vi "torres hanoi.vi"() -> ()   [LabVIEW 2020]
uses:
  <vilib>/Utility/miscctls.llb/LVPoint32TypeDef.ctl
  <vilib>/Utility/miscctls.llb/LVPositionTypeDef.ctl
  <vilib>/Utility/miscctls.llb/LVBoundsTypeDef.ctl
panel:
  out "Position 1":T1
  out "Position 2":T1
  out "Position 3":T1
  out "Position 4":T1
  out "Position 5":T1
  out "Position":T1
  in  "seleccione  numero de discos":u16(ring) items=["3"=3, "4"=4, "5"=5]
  out "Coords":T2
  in  "?":bool
  out "disco5":bool
  out "disco4":bool
  out "disco3":bool
  out "disco2":bool
  out "disco1":bool
  out "final":bool
  out "medio":bool
  out "inicio":bool
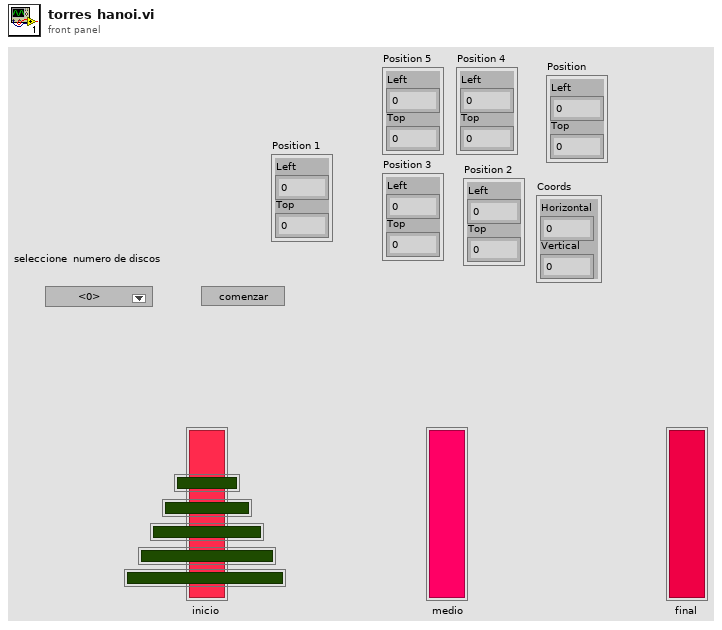
[diagram p1: front panel]
types:
  T1 = typedef "LVPositionTypeDef.ctl" = cluster{"Left":i32, "Top":i32}
  T2 = typedef "LVPoint32TypeDef.ctl" = cluster{"Horizontal":i32, "Vertical":i32}
  T3 = typedef "LVBoundsTypeDef.ctl" = cluster{"Width":u32, "Height":u32}
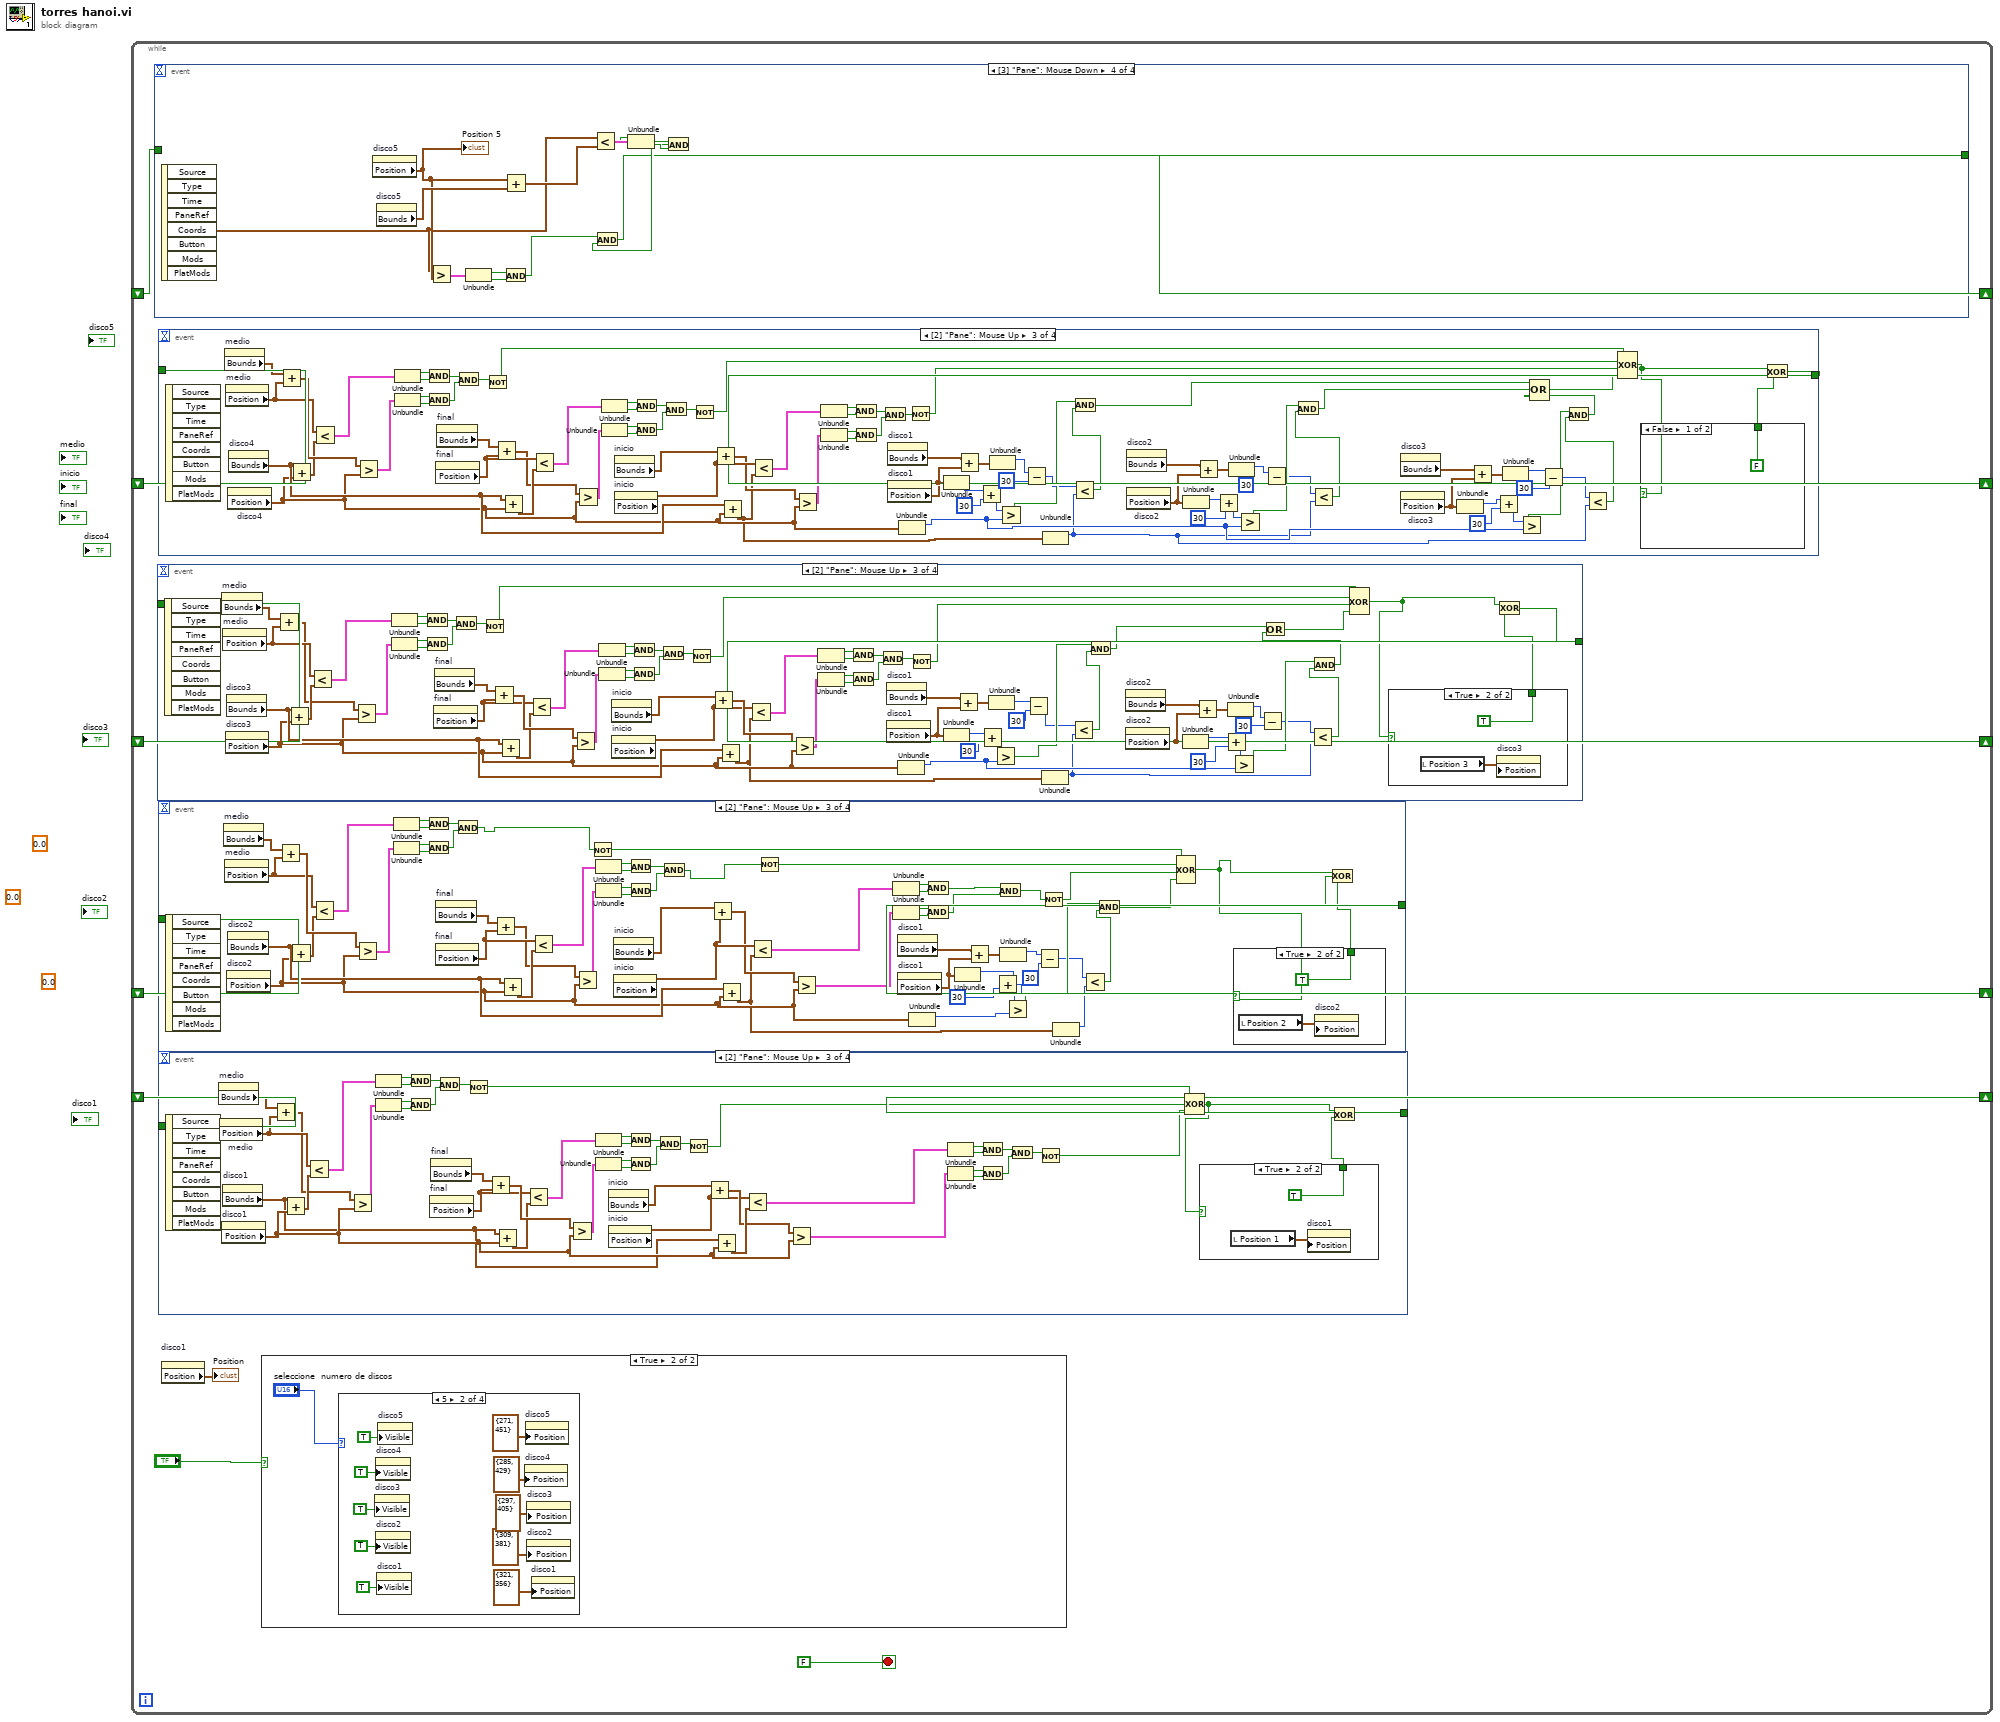
[diagram p0: block diagram]
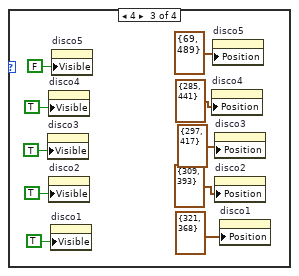
[diagram p4: hidden frame]
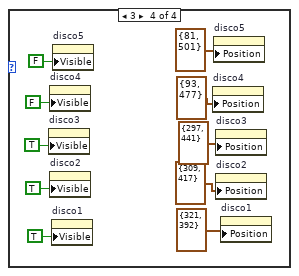
[diagram p5: hidden frame]
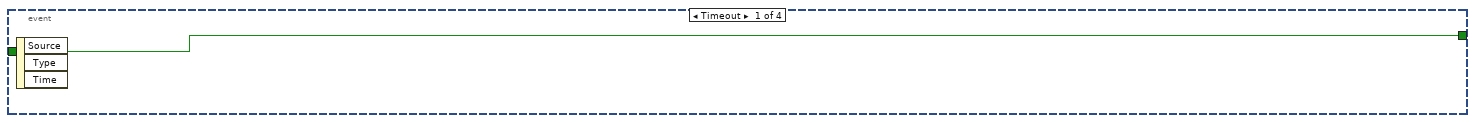
[diagram p6: hidden frame]
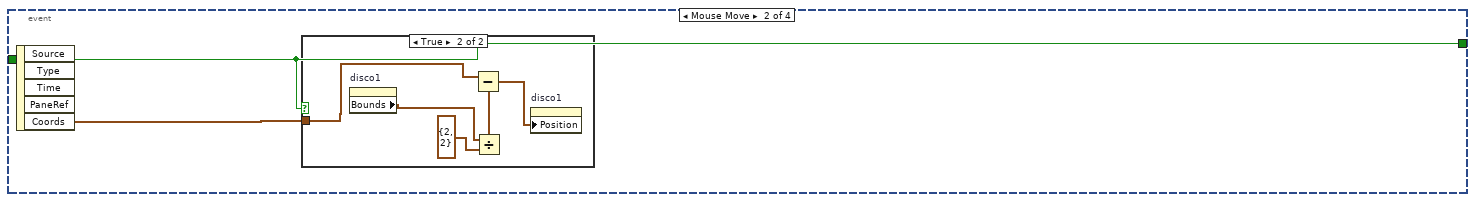
[diagram p7: hidden frame]
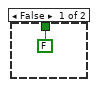
[diagram p9: hidden frame]
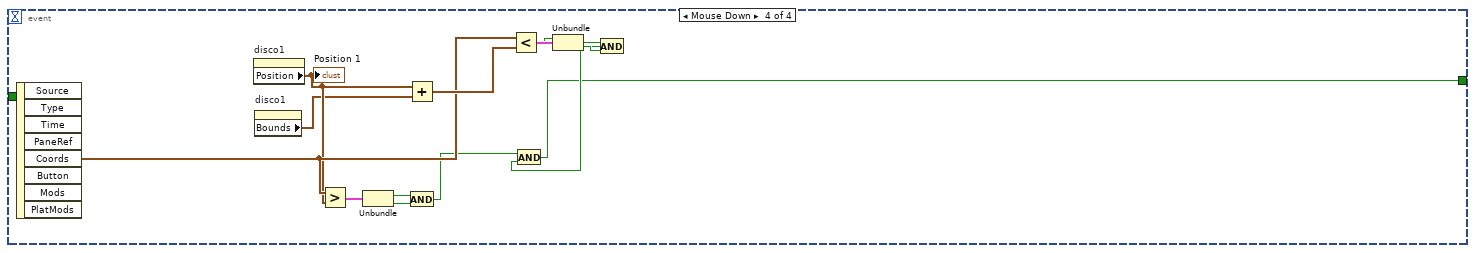
[diagram p10: hidden frame]
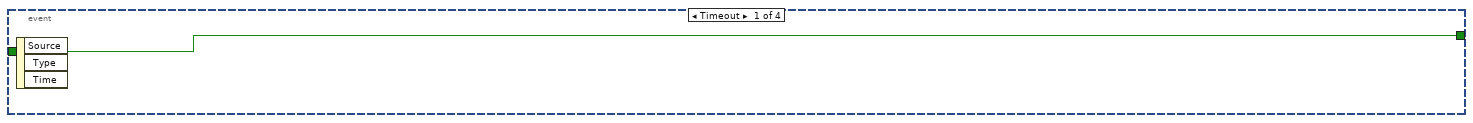
[diagram p11: hidden frame]
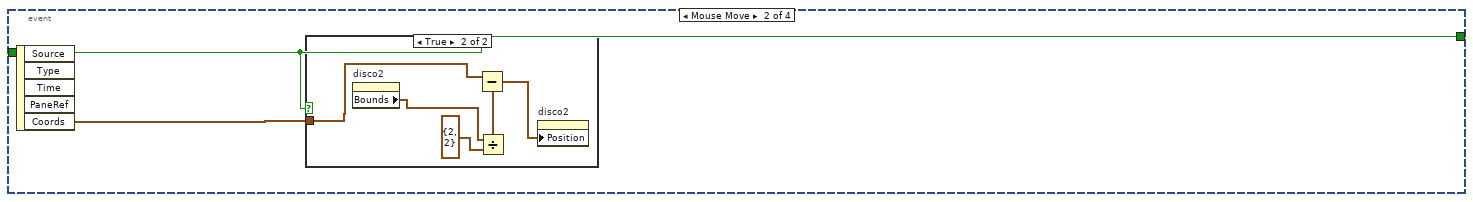
[diagram p12: hidden frame]
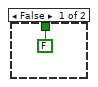
[diagram p14: hidden frame]
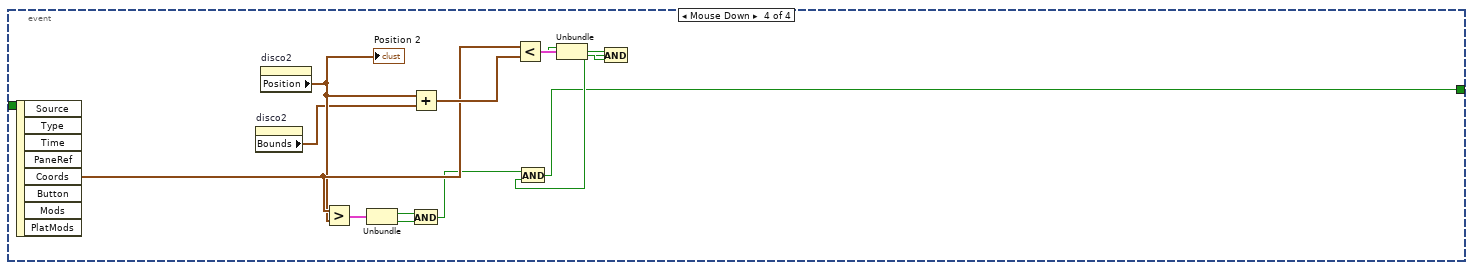
[diagram p15: hidden frame]
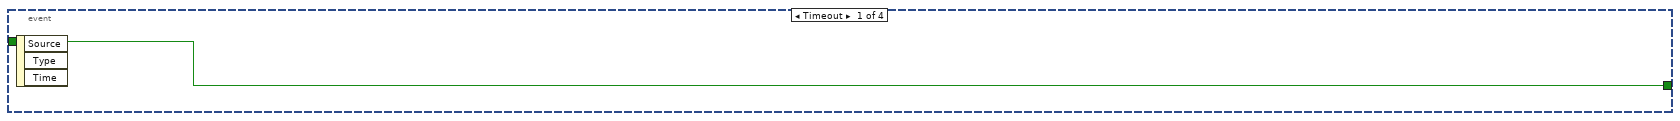
[diagram p16: hidden frame]
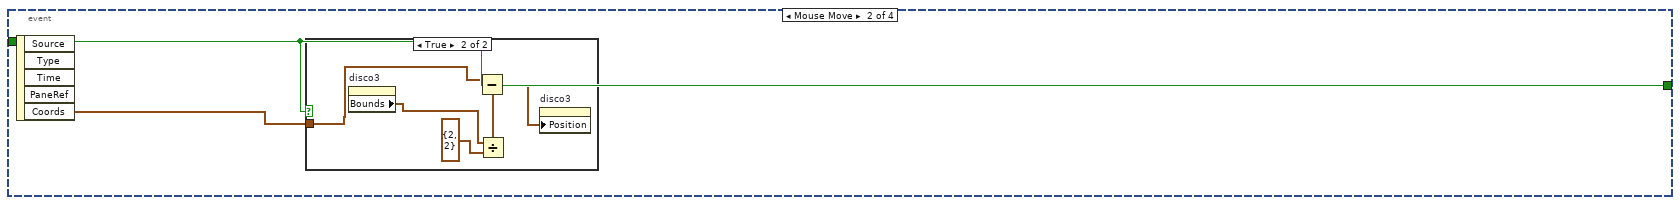
[diagram p17: hidden frame]
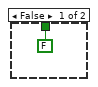
[diagram p19: hidden frame]
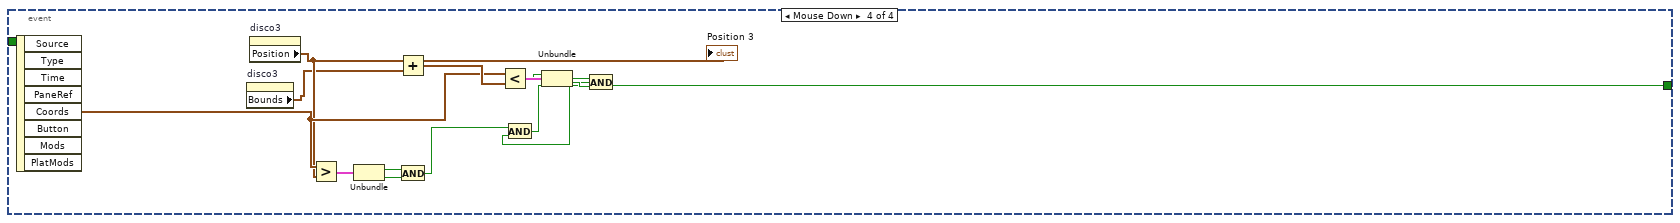
[diagram p20: hidden frame]
diagram:
  (unwired) 0.0 ("final b")
  (unwired) 0.0 ("inicio b")
  (unwired) 0.0 ("medio b")
  n1 = while {
    shift-right: [w11] -> _
    shift-left: _ -> [w12]
    shift-right: [w9] -> _
    shift-left: _ -> [w10]
    shift-right: [w7] -> _
    shift-left: _ -> [w8]
    shift-right: [w5] -> _
    shift-left: _ -> [w6]
    shift-right: [w3] -> _
    shift-left: _ -> [w4]
    stop <- FALSE stop-if-true
    n2 = event shown="[3] \"Pane\": Mouse Down" {
      selector: _ -> [_ _ _ _]
      dyn-events: _ -> [_ _ _ _]
      timeout: _ -> [_ _ _ _]
      tunnel: w12 -> [w409 w410 _ _]
      tunnel: [w409 w410 w470 w518] -> w11
      event Timeout {
        n3 = event-data() -> ()  [unwired: 1 in, 3 out]
      }
      event Mouse Move {
        n4 = event-data() -> ("Coords"=w411:T2)  [unwired: 1 in, 4 out]
        n5 = case shown="True" w410 {
          tunnel: w411 -> [_ w414]
          frame False {
          }
          frame True {
            n6 = property on="disco5" class="Bool (strict)"() -> ("Bounds"=w416:T3)  [unwired: 2 in, 2 out]
            n7 = Divide(x=w416, y=T3 {"Width"=2, "Height"=2}) -> (x/y=w413:cluster{"Width":dbl, "Height":dbl})
            n8 = Subtract(x=w414, y=w413) -> (x-y=w412:cluster{dbl, dbl})
            n9 = property on="disco5" class="Bool (strict)"("Position"=w412) -> ()  [unwired: 2 in, 2 out]
            "Coords" <- w414
          }
        }
      }
      event Mouse Up {
        n10 = event-data() -> ()  [unwired: 1 in, 8 out]
        n11 = property on="medio" class="Bool (strict)"() -> ("Bounds"=w505:T3)  [unwired: 2 in, 2 out]
        n12 = property on="medio" class="Bool (strict)"() -> ("Position"=w504:T1)  [unwired: 2 in, 2 out]
        n13 = property on="disco5" class="Bool (strict)"() -> ("Position"=w458:T1)  [unwired: 2 in, 2 out]
        n14 = property on="disco5" class="Bool (strict)"() -> ("Bounds"=w476:T3)  [unwired: 2 in, 2 out]
        n15 = Add(x=w505, y=w504) -> (x+y=w503:T3)
        n16 = Add(x=w476, y=w458) -> (x+y=w508:T3)
        n17 = Less?(x=w504, y=w508) -> (x < y?=w507:cluster{bool, bool})
        n18 = Greater?(x=w503, y=w458) -> (0:w506:cluster{bool, bool})
        n19 = Unbundle(w507) -> (w512:bool, w511:bool)
        n20 = Unbundle(w506) -> (w514:bool, w513:bool)
        n21 = And(x=w512, y=w511) -> (x .and. y?=w509:bool)
        n22 = And(x=w514, y=w513) -> (x .and. y?=w510:bool)
        n23 = property on="final" class="Bool (strict)"() -> ("Position"=w489:T1)  [unwired: 2 in, 2 out]
        n24 = property on="final" class="Bool (strict)"() -> ("Bounds"=w490:T3)  [unwired: 2 in, 2 out]
        n25 = And(x=w509, y=w510) -> (x .and. y?=w502:bool)
        n26 = Not(x=w502) -> (.not. x?=w473:bool)
        n27 = Add(x=w490, y=w489) -> (x+y=w500:T3)
        n28 = Add(x=w476, y=w458) -> (x+y=w497:T3)
        n29 = Less?(x=w489, y=w497) -> (x < y?=w498:cluster{bool, bool})
        n30 = Greater?(x=w500, y=w458) -> (0:w499:cluster{bool, bool})
        n31 = Unbundle(w498) -> (w493:bool, w494:bool)
        n32 = Unbundle(w499) -> (w491:bool, w492:bool)
        n33 = property on="inicio" class="Bool (strict)"() -> ("Bounds"=w478:T3)  [unwired: 2 in, 2 out]
        n34 = property on="inicio" class="Bool (strict)"() -> ("Position"=w477:T1)  [unwired: 2 in, 2 out]
        n35 = And(x=w493, y=w494) -> (x .and. y?=w496:bool)
        n36 = And(x=w491, y=w492) -> (x .and. y?=w495:bool)
        n37 = And(x=w496, y=w495) -> (x .and. y?=w501:bool)
        n38 = Not(x=w501) -> (.not. x?=w474:bool)
        n39 = Add(x=w478, y=w477) -> (x+y=w480:T3)
        n40 = Add(x=w476, y=w458) -> (x+y=w457:T3)
        n41 = Less?(x=w477, y=w457) -> (x < y?=w482:cluster{bool, bool})
        n42 = Greater?(x=w480, y=w458) -> (0:w481:cluster{bool, bool})
        n43 = Unbundle(w482) -> (w486:bool, w485:bool)
        n44 = Unbundle(w481) -> (w488:bool, w487:bool)
        n45 = property on="disco1" class="Bool (strict)"() -> ("Bounds"=w464:T3)  [unwired: 2 in, 2 out]
        n46 = property on="disco1" class="Bool (strict)"() -> ("Position"=w465:T1)  [unwired: 2 in, 2 out]
        n47 = Unbundle(w458) -> ("Left"=w447:i32)  [unwired: 1 out]
        n48 = And(x=w486, y=w485) -> (x .and. y?=w483:bool)
        n49 = And(x=w488, y=w487) -> (x .and. y?=w484:bool)
        n50 = And(x=w483, y=w484) -> (x .and. y?=w479:bool)
        n51 = Unbundle(w465) -> ("Left"=w445:i32)  [unwired: 1 out]
        n52 = Add(x=w464, y=w465) -> (x+y=w466:T3)
        n53 = Not(x=w479) -> (.not. x?=w475:bool)
        n54 = Add(x=w445, y=30) -> (x+y=w443:i32)
        n55 = Greater?(x=w443, y=w447) -> (0:w460:bool)
        n56 = Unbundle(w466) -> ("Width"=w442:u32)  [unwired: 1 out]
        n57 = Subtract(x=w442, y=u32 30) -> (x-y=w440:u32)
        n58 = Unbundle(w457) -> ("Width"=w446:u32)  [unwired: 1 out]
        n59 = Less?(x=w440, y=w446) -> (x < y?=w459:bool)
        n60 = And(x=w460, y=w459) -> (x .and. y?=w417:bool)
        n61 = property on="disco2" class="Bool (strict)"() -> ("Bounds"=w463:T3)  [unwired: 2 in, 2 out]
        n62 = property on="disco2" class="Bool (strict)"() -> ("Position"=w462:T1)  [unwired: 2 in, 2 out]
        n63 = Unbundle(w462) -> ("Left"=w438:i32)  [unwired: 1 out]
        n64 = Add(x=w463, y=w462) -> (x+y=w461:T3)
        n65 = Add(x=w438, y=30) -> (x+y=w439:i32)
        n66 = Unbundle(w461) -> ("Width"=w436:u32)  [unwired: 1 out]
        n67 = Greater?(x=w439, y=w447) -> (0:w456:bool)
        n68 = Subtract(x=w436, y=u32 30) -> (x-y=w435:u32)
        n69 = Less?(x=w435, y=w446) -> (x < y?=w455:bool)
        n70 = And(x=w456, y=w455) -> (x .and. y?=w418:bool)
        n71 = property on="disco3" class="Bool (strict)"() -> ("Bounds"=w467:T3)  [unwired: 2 in, 2 out]
        n72 = property on="disco3" class="Bool (strict)"() -> ("Position"=w468:T1)  [unwired: 2 in, 2 out]
        n73 = Unbundle(w468) -> ("Left"=w433:i32)  [unwired: 1 out]
        n74 = Add(x=w467, y=w468) -> (x+y=w469:T3)
        n75 = Add(x=w433, y=30) -> (x+y=w432:i32)
        n76 = Unbundle(w469) -> ("Width"=w430:u32)  [unwired: 1 out]
        n77 = Greater?(x=w432, y=w447) -> (0:w454:bool)
        n78 = Subtract(x=w430, y=u32 30) -> (x-y=w429:u32)
        n79 = Less?(x=w429, y=w446) -> (x < y?=w453:bool)
        n80 = And(x=w454, y=w453) -> (x .and. y?=w419:bool)
        n81 = property on="disco4" class="Bool (strict)"() -> ("Bounds"=w450:T3)  [unwired: 2 in, 2 out]
        n82 = property on="disco4" class="Bool (strict)"() -> ("Position"=w449:T1)  [unwired: 2 in, 2 out]
        n83 = Unbundle(w449) -> ("Left"=w427:i32)  [unwired: 1 out]
        n84 = Add(x=w450, y=w449) -> (x+y=w448:T3)
        n85 = Add(x=w427, y=30) -> (x+y=w426:i32)
        n86 = Greater?(x=w426, y=w447) -> (0:w451:bool)
        n87 = Unbundle(w448) -> ("Width"=w424:u32)  [unwired: 1 out]
        n88 = Subtract(x=w424, y=u32 30) -> (x-y=w422:u32)
        n89 = Less?(x=w422, y=w446) -> (x < y?=w452:bool)
        n90 = And(x=w451, y=w452) -> (x .and. y?=w420:bool)
        n91 = Compound Arithmetic op=OR(w417, w418, w419, w420) -> (w421:bool)
        n92 = Compound Arithmetic op=XOR(w473, w474, w475, w421) -> (w471:bool)
        n93 = case shown="True" w471 {
          tunnel: [FALSE ("Accepted?") TRUE ("Accepted?")] -> w472
          frame False {
          }
          frame True {
            n94 = local read "Position 5"() -> (w517:T1)
            n95 = property on="disco5" class="Bool (strict)"("Position"=w517) -> ()  [unwired: 2 in, 2 out]
          }
        }
        n96 = Exclusive Or(1:w472, 2:w471) -> (0:w470:bool)
      }
      event Mouse Down {
        n97 = event-data() -> ("Coords"=w527:T2)  [unwired: 1 in, 7 out]
        n98 = property on="disco5" class="Bool (strict)"() -> ("Position"=w529:T1)  [unwired: 2 in, 2 out]
        "Position 5" <- w529
        n99 = property on="disco5" class="Bool (strict)"() -> ("Bounds"=w530:T3)  [unwired: 2 in, 2 out]
        n100 = Greater?(x=w527, y=w529) -> (0:w526:cluster{bool, bool})
        n101 = Unbundle(w526) -> (w522:bool, w521:bool)
        n102 = Add(x=w529, y=w530) -> (x+y=w528:T3)
        n103 = And(x=w522, y=w521) -> (x .and. y?=w519:bool)
        n104 = Less?(x=w527, y=w528) -> (x < y?=w525:cluster{bool, bool})
        n105 = Unbundle(w525) -> (w524:bool, w523:bool)
        n106 = And(x=w524, y=w523) -> (x .and. y?=w520:bool)
        n107 = And(x=w519, y=w520) -> (x .and. y?=w518:bool)
      }
    }
    n108 = event shown="[2] \"Pane\": Mouse Up" {
      selector: _ -> [_ _ _ _]
      dyn-events: _ -> [_ _ _ _]
      timeout: _ -> [_ _ _ _]
      tunnel: w8 -> [w201 w202 _ _]
      tunnel: [w201 w202 w238 w288] -> w7
      event Timeout {
        n109 = event-data() -> ()  [unwired: 1 in, 3 out]
      }
      event Mouse Move {
        n110 = event-data() -> ("Coords"=w203:T2)  [unwired: 1 in, 4 out]
        n111 = case shown="True" w202 {
          tunnel: w203 -> [_ w207]
          frame False {
          }
          frame True {
            n112 = property on="disco3" class="Bool (strict)"() -> ("Bounds"=w205:T3)  [unwired: 2 in, 2 out]
            n113 = Divide(x=w205, y=T3 {"Width"=2, "Height"=2}) -> (x/y=w206:cluster{"Width":dbl, "Height":dbl})
            n114 = Subtract(x=w207, y=w206) -> (x-y=w204:cluster{dbl, dbl})
            n115 = property on="disco3" class="Bool (strict)"("Position"=w204) -> ()  [unwired: 2 in, 2 out]
          }
        }
      }
      event Mouse Up {
        n116 = event-data() -> ()  [unwired: 1 in, 8 out]
        n117 = property on="medio" class="Bool (strict)"() -> ("Bounds"=w273:T3)  [unwired: 2 in, 2 out]
        n118 = property on="medio" class="Bool (strict)"() -> ("Position"=w272:T1)  [unwired: 2 in, 2 out]
        n119 = property on="disco3" class="Bool (strict)"() -> ("Position"=w234:T1)  [unwired: 2 in, 2 out]
        n120 = property on="disco3" class="Bool (strict)"() -> ("Bounds"=w244:T3)  [unwired: 2 in, 2 out]
        n121 = Add(x=w273, y=w272) -> (x+y=w271:T3)
        n122 = Add(x=w244, y=w234) -> (x+y=w276:T3)
        n123 = Less?(x=w272, y=w276) -> (x < y?=w275:cluster{bool, bool})
        n124 = Greater?(x=w271, y=w234) -> (0:w274:cluster{bool, bool})
        n125 = Unbundle(w275) -> (w280:bool, w279:bool)
        n126 = Unbundle(w274) -> (w282:bool, w281:bool)
        n127 = And(x=w280, y=w279) -> (x .and. y?=w277:bool)
        n128 = And(x=w282, y=w281) -> (x .and. y?=w278:bool)
        n129 = property on="final" class="Bool (strict)"() -> ("Position"=w257:T1)  [unwired: 2 in, 2 out]
        n130 = property on="final" class="Bool (strict)"() -> ("Bounds"=w258:T3)  [unwired: 2 in, 2 out]
        n131 = And(x=w277, y=w278) -> (x .and. y?=w270:bool)
        n132 = Not(x=w270) -> (.not. x?=w241:bool)
        n133 = Add(x=w258, y=w257) -> (x+y=w268:T3)
        n134 = Add(x=w244, y=w234) -> (x+y=w265:T3)
        n135 = Less?(x=w257, y=w265) -> (x < y?=w266:cluster{bool, bool})
        n136 = Greater?(x=w268, y=w234) -> (0:w267:cluster{bool, bool})
        n137 = Unbundle(w266) -> (w261:bool, w262:bool)
        n138 = Unbundle(w267) -> (w259:bool, w260:bool)
        n139 = property on="inicio" class="Bool (strict)"() -> ("Bounds"=w246:T3)  [unwired: 2 in, 2 out]
        n140 = property on="inicio" class="Bool (strict)"() -> ("Position"=w245:T1)  [unwired: 2 in, 2 out]
        n141 = And(x=w261, y=w262) -> (x .and. y?=w264:bool)
        n142 = And(x=w259, y=w260) -> (x .and. y?=w263:bool)
        n143 = And(x=w264, y=w263) -> (x .and. y?=w269:bool)
        n144 = Not(x=w269) -> (.not. x?=w242:bool)
        n145 = Add(x=w246, y=w245) -> (x+y=w248:T3)
        n146 = Add(x=w244, y=w234) -> (x+y=w233:T3)
        n147 = Less?(x=w245, y=w233) -> (x < y?=w250:cluster{bool, bool})
        n148 = Greater?(x=w248, y=w234) -> (0:w249:cluster{bool, bool})
        n149 = Unbundle(w250) -> (w254:bool, w253:bool)
        n150 = Unbundle(w249) -> (w256:bool, w255:bool)
        n151 = And(x=w254, y=w253) -> (x .and. y?=w251:bool)
        n152 = And(x=w256, y=w255) -> (x .and. y?=w252:bool)
        n153 = And(x=w251, y=w252) -> (x .and. y?=w247:bool)
        n154 = property on="disco1" class="Bool (strict)"() -> ("Bounds"=w235:T3)  [unwired: 2 in, 2 out]
        n155 = property on="disco1" class="Bool (strict)"() -> ("Position"=w236:T1)  [unwired: 2 in, 2 out]
        n156 = Unbundle(w234) -> ("Left"=w227:i32)  [unwired: 1 out]
        n157 = Not(x=w247) -> (.not. x?=w243:bool)
        n158 = Unbundle(w236) -> ("Left"=w223:i32)  [unwired: 1 out]
        n159 = Add(x=w235, y=w236) -> (x+y=w237:T3)
        n160 = Add(x=w223, y=30) -> (x+y=w222:i32)
        n161 = Unbundle(w237) -> ("Width"=w219:u32)  [unwired: 1 out]
        n162 = Greater?(x=w222, y=w227) -> (0:w232:bool)
        n163 = Subtract(x=w219, y=u32 30) -> (x-y=w220:u32)
        n164 = Unbundle(w233) -> ("Width"=w226:u32)  [unwired: 1 out]
        n165 = Less?(x=w220, y=w226) -> (x < y?=w231:bool)
        n166 = And(x=w232, y=w231) -> (x .and. y?=w210:bool)
        n167 = property on="disco2" class="Bool (strict)"() -> ("Bounds"=w230:T3)  [unwired: 2 in, 2 out]
        n168 = property on="disco2" class="Bool (strict)"() -> ("Position"=w229:T1)  [unwired: 2 in, 2 out]
        n169 = Unbundle(w229) -> ("Left"=w217:i32)  [unwired: 1 out]
        n170 = Add(x=w230, y=w229) -> (x+y=w228:T3)
        n171 = Add(x=w217, y=30) -> (x+y=w216:i32)
        n172 = Unbundle(w228) -> ("Width"=w214:u32)  [unwired: 1 out]
        n173 = Greater?(x=w216, y=w227) -> (0:w224:bool)
        n174 = Subtract(x=w214, y=u32 30) -> (x-y=w213:u32)
        n175 = Less?(x=w213, y=w226) -> (x < y?=w225:bool)
        n176 = And(x=w224, y=w225) -> (x .and. y?=w211:bool)
        n177 = Or(x=w210, y=w211) -> (x .or. y?=w209:bool)
        n178 = Compound Arithmetic op=XOR(w241, w242, w243, w209) -> (w239:bool)
        n179 = case shown="True" w239 {
          tunnel: [FALSE ("Accepted?") TRUE ("Accepted?")] -> w240
          frame False {
          }
          frame True {
            n180 = local read "Position 3"() -> (w285:T1)
            n181 = property on="disco3" class="Bool (strict)"("Position"=w285) -> ()  [unwired: 2 in, 2 out]
          }
        }
        n182 = Exclusive Or(1:w240, 2:w239) -> (0:w238:bool)
      }
      event Mouse Down {
        n183 = event-data() -> ("Coords"=w297:T2)  [unwired: 1 in, 7 out]
        n184 = property on="disco3" class="Bool (strict)"() -> ("Bounds"=w286:T3)  [unwired: 2 in, 2 out]
        n185 = property on="disco3" class="Bool (strict)"() -> ("Position"=w287:T1)  [unwired: 2 in, 2 out]
        "Position 3" <- w287
        n186 = Greater?(x=w297, y=w287) -> (0:w296:cluster{bool, bool})
        n187 = Unbundle(w296) -> (w292:bool, w291:bool)
        n188 = Add(x=w287, y=w286) -> (x+y=w298:T3)
        n189 = And(x=w292, y=w291) -> (x .and. y?=w289:bool)
        n190 = Less?(x=w297, y=w298) -> (x < y?=w295:cluster{bool, bool})
        n191 = Unbundle(w295) -> (w294:bool, w293:bool)
        n192 = And(x=w294, y=w293) -> (x .and. y?=w290:bool)
        n193 = And(x=w289, y=w290) -> (x .and. y?=w288:bool)
      }
    }
    n194 = event shown="[2] \"Pane\": Mouse Up" {
      selector: _ -> [_ _ _ _]
      dyn-events: _ -> [_ _ _ _]
      timeout: _ -> [_ _ _ _]
      tunnel: w10 -> [w299 w300 _ _]
      tunnel: [w299 w300 w349 w398] -> w9
      event Timeout {
        n195 = event-data() -> ()  [unwired: 1 in, 3 out]
      }
      event Mouse Move {
        n196 = event-data() -> ("Coords"=w301:T2)  [unwired: 1 in, 4 out]
        n197 = case shown="True" w300 {
          tunnel: w301 -> [_ w302]
          frame False {
          }
          frame True {
            n198 = property on="disco4" class="Bool (strict)"() -> ("Bounds"=w304:T3)  [unwired: 2 in, 2 out]
            n199 = Divide(x=w304, y=T3 {"Width"=2, "Height"=2}) -> (x/y=w305:cluster{"Width":dbl, "Height":dbl})
            n200 = Subtract(x=w302, y=w305) -> (x-y=w303:cluster{dbl, dbl})
            n201 = property on="disco4" class="Bool (strict)"("Position"=w303) -> ()  [unwired: 2 in, 2 out]
          }
        }
      }
      event Mouse Up {
        n202 = event-data() -> ()  [unwired: 1 in, 8 out]
        n203 = property on="medio" class="Bool (strict)"() -> ("Bounds"=w359:T3)  [unwired: 2 in, 2 out]
        n204 = property on="medio" class="Bool (strict)"() -> ("Position"=w360:T1)  [unwired: 2 in, 2 out]
        n205 = property on="disco4" class="Bool (strict)"() -> ("Position"=w338:T1)  [unwired: 2 in, 2 out]
        n206 = property on="disco4" class="Bool (strict)"() -> ("Bounds"=w388:T3)  [unwired: 2 in, 2 out]
        n207 = Add(x=w359, y=w360) -> (x+y=w361:T3)
        n208 = Add(x=w388, y=w338) -> (x+y=w356:T3)
        n209 = Less?(x=w360, y=w356) -> (x < y?=w357:cluster{bool, bool})
        n210 = Greater?(x=w361, y=w338) -> (0:w358:cluster{bool, bool})
        n211 = Unbundle(w357) -> (w352:bool, w353:bool)
        n212 = Unbundle(w358) -> (w350:bool, w351:bool)
        n213 = And(x=w352, y=w353) -> (x .and. y?=w355:bool)
        n214 = And(x=w350, y=w351) -> (x .and. y?=w354:bool)
        n215 = property on="final" class="Bool (strict)"() -> ("Position"=w375:T1)  [unwired: 2 in, 2 out]
        n216 = property on="final" class="Bool (strict)"() -> ("Bounds"=w374:T3)  [unwired: 2 in, 2 out]
        n217 = And(x=w355, y=w354) -> (x .and. y?=w362:bool)
        n218 = Not(x=w362) -> (.not. x?=w390:bool)
        n219 = Add(x=w374, y=w375) -> (x+y=w364:T3)
        n220 = Add(x=w388, y=w338) -> (x+y=w367:T3)
        n221 = Less?(x=w375, y=w367) -> (x < y?=w366:cluster{bool, bool})
        n222 = Greater?(x=w364, y=w338) -> (0:w365:cluster{bool, bool})
        n223 = Unbundle(w366) -> (w371:bool, w370:bool)
        n224 = Unbundle(w365) -> (w373:bool, w372:bool)
        n225 = property on="inicio" class="Bool (strict)"() -> ("Bounds"=w386:T3)  [unwired: 2 in, 2 out]
        n226 = property on="inicio" class="Bool (strict)"() -> ("Position"=w387:T1)  [unwired: 2 in, 2 out]
        n227 = And(x=w371, y=w370) -> (x .and. y?=w368:bool)
        n228 = And(x=w373, y=w372) -> (x .and. y?=w369:bool)
        n229 = And(x=w368, y=w369) -> (x .and. y?=w363:bool)
        n230 = Not(x=w363) -> (.not. x?=w389:bool)
        n231 = Add(x=w386, y=w387) -> (x+y=w384:T3)
        n232 = Add(x=w388, y=w338) -> (x+y=w337:T3)
        n233 = Less?(x=w387, y=w337) -> (x < y?=w382:cluster{bool, bool})
        n234 = Greater?(x=w384, y=w338) -> (0:w383:cluster{bool, bool})
        n235 = Unbundle(w382) -> (w378:bool, w379:bool)
        n236 = Unbundle(w383) -> (w376:bool, w377:bool)
        n237 = And(x=w378, y=w379) -> (x .and. y?=w381:bool)
        n238 = And(x=w376, y=w377) -> (x .and. y?=w380:bool)
        n239 = And(x=w381, y=w380) -> (x .and. y?=w385:bool)
        n240 = property on="disco1" class="Bool (strict)"() -> ("Bounds"=w345:T3)  [unwired: 2 in, 2 out]
        n241 = property on="disco1" class="Bool (strict)"() -> ("Position"=w344:T1)  [unwired: 2 in, 2 out]
        n242 = Unbundle(w338) -> ("Left"=w333:i32)  [unwired: 1 out]
        n243 = Not(x=w385) -> (.not. x?=w308:bool)
        n244 = Unbundle(w344) -> ("Left"=w329:i32)  [unwired: 1 out]
        n245 = Add(x=w345, y=w344) -> (x+y=w343:T3)
        n246 = Add(x=w329, y=30) -> (x+y=w327:i32)
        n247 = Unbundle(w343) -> ("Width"=w326:u32)  [unwired: 1 out]
        n248 = Greater?(x=w327, y=w333) -> (0:w340:bool)
        n249 = Subtract(x=w326, y=u32 30) -> (x-y=w325:u32)
        n250 = Unbundle(w337) -> ("Width"=w332:u32)  [unwired: 1 out]
        n251 = Less?(x=w325, y=w332) -> (x < y?=w339:bool)
        n252 = And(x=w340, y=w339) -> (x .and. y?=w309:bool)
        n253 = property on="disco2" class="Bool (strict)"() -> ("Bounds"=w346:T3)  [unwired: 2 in, 2 out]
        n254 = property on="disco2" class="Bool (strict)"() -> ("Position"=w347:T1)  [unwired: 2 in, 2 out]
        n255 = Unbundle(w347) -> ("Left"=w322:i32)  [unwired: 1 out]
        n256 = Add(x=w346, y=w347) -> (x+y=w348:T3)
        n257 = Add(x=w322, y=30) -> (x+y=w323:i32)
        n258 = Unbundle(w348) -> ("Width"=w320:u32)  [unwired: 1 out]
        n259 = Greater?(x=w323, y=w333) -> (0:w342:bool)
        n260 = Subtract(x=w320, y=u32 30) -> (x-y=w318:u32)
        n261 = Less?(x=w318, y=w332) -> (x < y?=w341:bool)
        n262 = And(x=w342, y=w341) -> (x .and. y?=w310:bool)
        n263 = property on="disco3" class="Bool (strict)"() -> ("Bounds"=w336:T3)  [unwired: 2 in, 2 out]
        n264 = property on="disco3" class="Bool (strict)"() -> ("Position"=w335:T1)  [unwired: 2 in, 2 out]
        n265 = Unbundle(w335) -> ("Left"=w317:i32)  [unwired: 1 out]
        n266 = Add(x=w336, y=w335) -> (x+y=w334:T3)
        n267 = Add(x=w317, y=30) -> (x+y=w316:i32)
        n268 = Unbundle(w334) -> ("Width"=w314:u32)  [unwired: 1 out]
        n269 = Greater?(x=w316, y=w333) -> (0:w331:bool)
        n270 = Subtract(x=w314, y=u32 30) -> (x-y=w313:u32)
        n271 = Less?(x=w313, y=w332) -> (x < y?=w330:bool)
        n272 = And(x=w331, y=w330) -> (x .and. y?=w311:bool)
        n273 = Compound Arithmetic op=OR(w309, w310, w311) -> (w307:bool)
        n274 = Compound Arithmetic op=XOR(w390, w389, w308, w307) -> (w392:bool)
        n275 = case shown="False" w392 {
          tunnel: [FALSE ("Accepted?") TRUE ("Accepted?")] -> w391
          frame False {
          }
          frame True {
            n276 = local read "Position 4"() -> (w395:T1)
            n277 = property on="disco4" class="Bool (strict)"("Position"=w395) -> ()  [unwired: 2 in, 2 out]
          }
        }
        n278 = Exclusive Or(1:w391, 2:w392) -> (0:w349:bool)
      }
      event Mouse Down {
        n279 = event-data() -> ("Coords"=w407:T2)  [unwired: 1 in, 7 out]
        n280 = property on="disco4" class="Bool (strict)"() -> ("Position"=w397:T1)  [unwired: 2 in, 2 out]
        "Position 4" <- w397
        n281 = property on="disco4" class="Bool (strict)"() -> ("Bounds"=w396:T3)  [unwired: 2 in, 2 out]
        n282 = Greater?(x=w407, y=w397) -> (0:w406:cluster{bool, bool})
        n283 = Unbundle(w406) -> (w402:bool, w401:bool)
        n284 = Add(x=w397, y=w396) -> (x+y=w408:T3)
        n285 = And(x=w402, y=w401) -> (x .and. y?=w399:bool)
        n286 = Less?(x=w407, y=w408) -> (x < y?=w405:cluster{bool, bool})
        n287 = Unbundle(w405) -> (w404:bool, w403:bool)
        n288 = And(x=w404, y=w403) -> (x .and. y?=w400:bool)
        n289 = And(x=w399, y=w400) -> (x .and. y?=w398:bool)
      }
    }
    n290 = event shown="[2] \"Pane\": Mouse Up" {
      selector: _ -> [_ _ _ _]
      dyn-events: _ -> [_ _ _ _]
      timeout: _ -> [_ _ _ _]
      tunnel: w6 -> [w116 w117 _ _]
      tunnel: [w116 w117 w144 w190] -> w5
      event Timeout {
        n291 = event-data() -> ()  [unwired: 1 in, 3 out]
      }
      event Mouse Move {
        n292 = event-data() -> ("Coords"=w118:T2)  [unwired: 1 in, 4 out]
        n293 = case shown="True" w117 {
          tunnel: w118 -> [_ w122]
          frame False {
          }
          frame True {
            n294 = property on="disco2" class="Bool (strict)"() -> ("Bounds"=w120:T3)  [unwired: 2 in, 2 out]
            n295 = Divide(x=w120, y=T3 {"Width"=2, "Height"=2}) -> (x/y=w121:cluster{"Width":dbl, "Height":dbl})
            n296 = Subtract(x=w122, y=w121) -> (x-y=w119:cluster{dbl, dbl})
            n297 = property on="disco2" class="Bool (strict)"("Position"=w119) -> ()  [unwired: 2 in, 2 out]
          }
        }
      }
      event Mouse Up {
        n298 = event-data() -> ()  [unwired: 1 in, 8 out]
        n299 = property on="medio" class="Bool (strict)"() -> ("Bounds"=w154:T3)  [unwired: 2 in, 2 out]
        n300 = property on="medio" class="Bool (strict)"() -> ("Position"=w155:T1)  [unwired: 2 in, 2 out]
        n301 = property on="disco2" class="Bool (strict)"() -> ("Position"=w139:T1)  [unwired: 2 in, 2 out]
        n302 = property on="disco2" class="Bool (strict)"() -> ("Bounds"=w180:T3)  [unwired: 2 in, 2 out]
        n303 = Add(x=w154, y=w155) -> (x+y=w156:T3)
        n304 = Add(x=w180, y=w139) -> (x+y=w151:T3)
        n305 = Less?(x=w155, y=w151) -> (x < y?=w152:cluster{bool, bool})
        n306 = Greater?(x=w156, y=w139) -> (0:w153:cluster{bool, bool})
        n307 = Unbundle(w152) -> (w147:bool, w148:bool)
        n308 = Unbundle(w153) -> (w145:bool, w146:bool)
        n309 = And(x=w147, y=w148) -> (x .and. y?=w150:bool)
        n310 = And(x=w145, y=w146) -> (x .and. y?=w149:bool)
        n311 = property on="final" class="Bool (strict)"() -> ("Position"=w168:T1)  [unwired: 2 in, 2 out]
        n312 = property on="final" class="Bool (strict)"() -> ("Bounds"=w167:T3)  [unwired: 2 in, 2 out]
        n313 = And(x=w150, y=w149) -> (x .and. y?=w142:bool)
        n314 = Add(x=w167, y=w168) -> (x+y=w157:T3)
        n315 = Add(x=w180, y=w139) -> (x+y=w160:T3)
        n316 = Less?(x=w168, y=w160) -> (x < y?=w159:cluster{bool, bool})
        n317 = Greater?(x=w157, y=w139) -> (0:w158:cluster{bool, bool})
        n318 = Not(x=w142) -> (.not. x?=w182:bool)
        n319 = Unbundle(w159) -> (w164:bool, w163:bool)
        n320 = Unbundle(w158) -> (w166:bool, w165:bool)
        n321 = property on="inicio" class="Bool (strict)"() -> ("Bounds"=w178:T3)  [unwired: 2 in, 2 out]
        n322 = property on="inicio" class="Bool (strict)"() -> ("Position"=w179:T1)  [unwired: 2 in, 2 out]
        n323 = And(x=w164, y=w163) -> (x .and. y?=w161:bool)
        n324 = And(x=w166, y=w165) -> (x .and. y?=w162:bool)
        n325 = And(x=w161, y=w162) -> (x .and. y?=w141:bool)
        n326 = Add(x=w178, y=w179) -> (x+y=w177:T3)
        n327 = Add(x=w180, y=w139) -> (x+y=w135:T3)
        n328 = Less?(x=w179, y=w135) -> (x < y?=w175:cluster{bool, bool})
        n329 = Not(x=w141) -> (.not. x?=w143:bool)
        n330 = Greater?(x=w177, y=w139) -> (0:w176:cluster{bool, bool})
        n331 = Unbundle(w175) -> (w171:bool, w172:bool)
        n332 = Unbundle(w176) -> (w169:bool, w170:bool)
        n333 = property on="disco1" class="Bool (strict)"() -> ("Bounds"=w138:T3)  [unwired: 2 in, 2 out]
        n334 = property on="disco1" class="Bool (strict)"() -> ("Position"=w137:T1)  [unwired: 2 in, 2 out]
        n335 = Unbundle(w139) -> ("Left"=w130:i32)  [unwired: 1 out]
        n336 = And(x=w171, y=w172) -> (x .and. y?=w174:bool)
        n337 = And(x=w169, y=w170) -> (x .and. y?=w173:bool)
        n338 = Unbundle(w137) -> ("Left"=w129:i32)  [unwired: 1 out]
        n339 = Add(x=w138, y=w137) -> (x+y=w136:T3)
        n340 = Add(x=w129, y=30) -> (x+y=w127:i32)
        n341 = And(x=w174, y=w173) -> (x .and. y?=w140:bool)
        n342 = Unbundle(w136) -> ("Width"=w125:u32)  [unwired: 1 out]
        n343 = Greater?(x=w127, y=w130) -> (0:w133:bool)
        n344 = Subtract(x=w125, y=u32 30) -> (x-y=w126:u32)
        n345 = Not(x=w140) -> (.not. x?=w181:bool)
        n346 = Unbundle(w135) -> ("Width"=w134:u32)  [unwired: 1 out]
        n347 = Less?(x=w126, y=w134) -> (x < y?=w132:bool)
        n348 = And(x=w133, y=w132) -> (x .and. y?=w131:bool)
        n349 = Compound Arithmetic op=XOR(w182, w143, w181, w131) -> (w184:bool)
        n350 = case shown="True" w184 {
          tunnel: [FALSE ("Accepted?") TRUE ("Accepted?")] -> w183
          frame False {
          }
          frame True {
            n351 = local read "Position 2"() -> (w187:T1)
            n352 = property on="disco2" class="Bool (strict)"("Position"=w187) -> ()  [unwired: 2 in, 2 out]
          }
        }
        n353 = Exclusive Or(1:w183, 2:w184) -> (0:w144:bool)
      }
      event Mouse Down {
        n354 = event-data() -> ("Coords"=w199:T2)  [unwired: 1 in, 7 out]
        n355 = property on="disco2" class="Bool (strict)"() -> ("Bounds"=w188:T3)  [unwired: 2 in, 2 out]
        n356 = property on="disco2" class="Bool (strict)"() -> ("Position"=w189:T1)  [unwired: 2 in, 2 out]
        "Position 2" <- w189
        n357 = Greater?(x=w199, y=w189) -> (0:w198:cluster{bool, bool})
        n358 = Unbundle(w198) -> (w194:bool, w193:bool)
        n359 = Add(x=w189, y=w188) -> (x+y=w200:T3)
        n360 = And(x=w194, y=w193) -> (x .and. y?=w191:bool)
        n361 = Less?(x=w199, y=w200) -> (x < y?=w197:cluster{bool, bool})
        n362 = Unbundle(w197) -> (w196:bool, w195:bool)
        n363 = And(x=w196, y=w195) -> (x .and. y?=w192:bool)
        n364 = And(x=w191, y=w192) -> (x .and. y?=w190:bool)
      }
    }
    n365 = event shown="[2] \"Pane\": Mouse Up" {
      selector: _ -> [_ _ _ _]
      dyn-events: _ -> [_ _ _ _]
      timeout: _ -> [_ _ _ _]
      tunnel: w4 -> [w45 w46 _ _]
      tunnel: [w45 w46 w56 w105] -> w3
      event Timeout {
        n366 = event-data() -> ()  [unwired: 1 in, 3 out]
      }
      event Mouse Move {
        n367 = event-data() -> ("Coords"=w47:T2)  [unwired: 1 in, 4 out]
        n368 = case shown="True" w46 {
          tunnel: w47 -> [_ w51]
          frame False {
          }
          frame True {
            n369 = property on="disco1" class="Bool (strict)"() -> ("Bounds"=w49:T3)  [unwired: 2 in, 2 out]
            n370 = Divide(x=w49, y=T3 {"Width"=2, "Height"=2}) -> (x/y=w50:cluster{"Width":dbl, "Height":dbl})
            n371 = Subtract(x=w51, y=w50) -> (x-y=w48:cluster{dbl, dbl})
            n372 = property on="disco1" class="Bool (strict)"("Position"=w48) -> ()  [unwired: 2 in, 2 out]
          }
        }
      }
      event Mouse Up {
        n373 = event-data() -> ()  [unwired: 1 in, 8 out]
        n374 = property on="medio" class="Bool (strict)"() -> ("Bounds"=w90:T3)  [unwired: 2 in, 2 out]
        n375 = property on="medio" class="Bool (strict)"() -> ("Position"=w89:T1)  [unwired: 2 in, 2 out]
        n376 = property on="disco1" class="Bool (strict)"() -> ("Position"=w63:T1)  [unwired: 2 in, 2 out]
        n377 = property on="disco1" class="Bool (strict)"() -> ("Bounds"=w62:T3)  [unwired: 2 in, 2 out]
        n378 = Add(x=w90, y=w89) -> (x+y=w88:T3)
        n379 = Add(x=w62, y=w63) -> (x+y=w93:T3)
        n380 = Less?(x=w89, y=w93) -> (x < y?=w92:cluster{bool, bool})
        n381 = Greater?(x=w88, y=w63) -> (0:w91:cluster{bool, bool})
        n382 = Unbundle(w92) -> (w97:bool, w96:bool)
        n383 = Unbundle(w91) -> (w99:bool, w98:bool)
        n384 = And(x=w97, y=w96) -> (x .and. y?=w94:bool)
        n385 = And(x=w99, y=w98) -> (x .and. y?=w95:bool)
        n386 = property on="final" class="Bool (strict)"() -> ("Position"=w76:T1)  [unwired: 2 in, 2 out]
        n387 = property on="final" class="Bool (strict)"() -> ("Bounds"=w77:T3)  [unwired: 2 in, 2 out]
        n388 = And(x=w94, y=w95) -> (x .and. y?=w55:bool)
        n389 = Not(x=w55) -> (.not. x?=w59:bool)
        n390 = Add(x=w77, y=w76) -> (x+y=w87:T3)
        n391 = Add(x=w62, y=w63) -> (x+y=w84:T3)
        n392 = Less?(x=w76, y=w84) -> (x < y?=w85:cluster{bool, bool})
        n393 = Greater?(x=w87, y=w63) -> (0:w86:cluster{bool, bool})
        n394 = Unbundle(w85) -> (w80:bool, w81:bool)
        n395 = Unbundle(w86) -> (w78:bool, w79:bool)
        n396 = property on="inicio" class="Bool (strict)"() -> ("Bounds"=w65:T3)  [unwired: 2 in, 2 out]
        n397 = property on="inicio" class="Bool (strict)"() -> ("Position"=w64:T1)  [unwired: 2 in, 2 out]
        n398 = And(x=w80, y=w81) -> (x .and. y?=w83:bool)
        n399 = And(x=w78, y=w79) -> (x .and. y?=w82:bool)
        n400 = And(x=w83, y=w82) -> (x .and. y?=w54:bool)
        n401 = Not(x=w54) -> (.not. x?=w60:bool)
        n402 = Add(x=w65, y=w64) -> (x+y=w66:T3)
        n403 = Add(x=w62, y=w63) -> (x+y=w69:T3)
        n404 = Less?(x=w64, y=w69) -> (x < y?=w68:cluster{bool, bool})
        n405 = Greater?(x=w66, y=w63) -> (0:w67:cluster{bool, bool})
        n406 = Unbundle(w68) -> (w73:bool, w72:bool)
        n407 = Unbundle(w67) -> (w75:bool, w74:bool)
        n408 = And(x=w73, y=w72) -> (x .and. y?=w70:bool)
        n409 = And(x=w75, y=w74) -> (x .and. y?=w71:bool)
        n410 = And(x=w70, y=w71) -> (x .and. y?=w53:bool)
        n411 = Not(x=w53) -> (.not. x?=w61:bool)
        n412 = Compound Arithmetic op=XOR(w59, w60, w61) -> (w58:bool)
        n413 = case shown="True" w58 {
          tunnel: [FALSE ("Accepted?") TRUE ("Accepted?")] -> w57
          frame False {
          }
          frame True {
            n414 = local read "Position 1"() -> (w102:T1)
            n415 = property on="disco1" class="Bool (strict)"("Position"=w102) -> ()  [unwired: 2 in, 2 out]
          }
        }
        n416 = Exclusive Or(1:w57, 2:w58) -> (0:w56:bool)
      }
      event Mouse Down {
        n417 = event-data() -> ("Coords"=w114:T2)  [unwired: 1 in, 7 out]
        n418 = property on="disco1" class="Bool (strict)"() -> ("Position"=w104:T1)  [unwired: 2 in, 2 out]
        "Position 1" <- w104
        n419 = property on="disco1" class="Bool (strict)"() -> ("Bounds"=w103:T3)  [unwired: 2 in, 2 out]
        n420 = Greater?(x=w114, y=w104) -> (0:w113:cluster{bool, bool})
        n421 = Unbundle(w113) -> (w109:bool, w108:bool)
        n422 = Add(x=w104, y=w103) -> (x+y=w115:T3)
        n423 = And(x=w109, y=w108) -> (x .and. y?=w106:bool)
        n424 = Less?(x=w114, y=w115) -> (x < y?=w112:cluster{bool, bool})
        n425 = Unbundle(w112) -> (w111:bool, w110:bool)
        n426 = And(x=w111, y=w110) -> (x .and. y?=w107:bool)
        n427 = And(x=w106, y=w107) -> (x .and. y?=w105:bool)
      }
    }
    n428 = property on="disco1" class="Bool (strict)"() -> ("Position"=→"Position":T1)  [unwired: 2 in, 2 out]
    n429 = case shown="True" "?" {
      frame False {
      }
      frame True {
        n430 = case shown="5" "seleccione  numero de discos" {
          frame 0, Default {
          }
          frame 5 {
            n431 = property on="disco3" class="Bool (strict)"("Visible"=TRUE) -> ()  [unwired: 2 in, 2 out]
            n432 = property on="disco4" class="Bool (strict)"("Visible"=TRUE) -> ()  [unwired: 2 in, 2 out]
            n433 = property on="disco2" class="Bool (strict)"("Visible"=TRUE) -> ()  [unwired: 2 in, 2 out]
            n434 = property on="disco1" class="Bool (strict)"("Visible"=TRUE) -> ()  [unwired: 2 in, 2 out]
            n435 = property on="disco5" class="Bool (strict)"("Visible"=TRUE) -> ()  [unwired: 2 in, 2 out]
            n436 = property on="disco4" class="Bool (strict)"("Position"=T1 {"Left"=285, "Top"=429}) -> ()  [unwired: 2 in, 2 out]
            n437 = property on="disco5" class="Bool (strict)"("Position"=T1 {"Left"=271, "Top"=451}) -> ()  [unwired: 2 in, 2 out]
            n438 = property on="disco3" class="Bool (strict)"("Position"=T1 {"Left"=297, "Top"=405}) -> ()  [unwired: 2 in, 2 out]
            n439 = property on="disco2" class="Bool (strict)"("Position"=T1 {"Left"=309, "Top"=381}) -> ()  [unwired: 2 in, 2 out]
            n440 = property on="disco1" class="Bool (strict)"("Position"=T1 {"Left"=321, "Top"=356}) -> ()  [unwired: 2 in, 2 out]
          }
          frame 4 {
            n441 = property on="disco3" class="Bool (strict)"("Visible"=TRUE) -> ()  [unwired: 2 in, 2 out]
            n442 = property on="disco4" class="Bool (strict)"("Visible"=TRUE) -> ()  [unwired: 2 in, 2 out]
            n443 = property on="disco2" class="Bool (strict)"("Visible"=TRUE) -> ()  [unwired: 2 in, 2 out]
            n444 = property on="disco1" class="Bool (strict)"("Visible"=TRUE) -> ()  [unwired: 2 in, 2 out]
            n445 = property on="disco5" class="Bool (strict)"("Visible"=FALSE) -> ()  [unwired: 2 in, 2 out]
            n446 = property on="disco4" class="Bool (strict)"("Position"=T1 {"Left"=285, "Top"=441}) -> ()  [unwired: 2 in, 2 out]
            n447 = property on="disco5" class="Bool (strict)"("Position"=T1 {"Left"=69, "Top"=489}) -> ()  [unwired: 2 in, 2 out]
            n448 = property on="disco3" class="Bool (strict)"("Position"=T1 {"Left"=297, "Top"=417}) -> ()  [unwired: 2 in, 2 out]
            n449 = property on="disco2" class="Bool (strict)"("Position"=T1 {"Left"=309, "Top"=393}) -> ()  [unwired: 2 in, 2 out]
            n450 = property on="disco1" class="Bool (strict)"("Position"=T1 {"Left"=321, "Top"=368}) -> ()  [unwired: 2 in, 2 out]
          }
          frame 3 {
            n451 = property on="disco3" class="Bool (strict)"("Visible"=TRUE) -> ()  [unwired: 2 in, 2 out]
            n452 = property on="disco4" class="Bool (strict)"("Visible"=FALSE) -> ()  [unwired: 2 in, 2 out]
            n453 = property on="disco2" class="Bool (strict)"("Visible"=TRUE) -> ()  [unwired: 2 in, 2 out]
            n454 = property on="disco1" class="Bool (strict)"("Visible"=TRUE) -> ()  [unwired: 2 in, 2 out]
            n455 = property on="disco5" class="Bool (strict)"("Visible"=FALSE) -> ()  [unwired: 2 in, 2 out]
            n456 = property on="disco4" class="Bool (strict)"("Position"=T1 {"Left"=93, "Top"=477}) -> ()  [unwired: 2 in, 2 out]
            n457 = property on="disco5" class="Bool (strict)"("Position"=T1 {"Left"=81, "Top"=501}) -> ()  [unwired: 2 in, 2 out]
            n458 = property on="disco3" class="Bool (strict)"("Position"=T1 {"Left"=297, "Top"=441}) -> ()  [unwired: 2 in, 2 out]
            n459 = property on="disco2" class="Bool (strict)"("Position"=T1 {"Left"=309, "Top"=417}) -> ()  [unwired: 2 in, 2 out]
            n460 = property on="disco1" class="Bool (strict)"("Position"=T1 {"Left"=321, "Top"=392}) -> ()  [unwired: 2 in, 2 out]
          }
        }
      }
    }
  }
